vi "InjectApplicationReference.vi"(8 "error in (no error)":errorcluster, 10 "Application":refnum<vi>, 11 "CreateClass In":refnum<class "CreateClass.lvclass">) -> (0 "error out":errorcluster, 3 "CreateClass Out":refnum<class "CreateClass.lvclass">)   [LabVIEW 2020, in "Mermaid.lvlib" / "CreateClass.lvclass"]
uses:
  CreateClass.lvclass
  CreateClass.lvclass/CreateClass.ctl
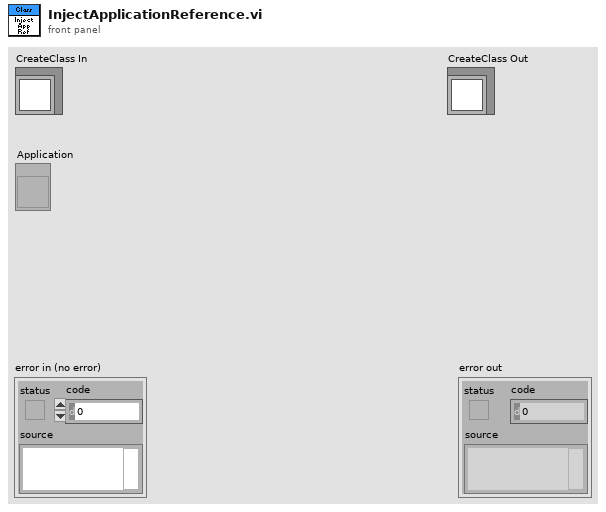
[diagram p1: front panel]
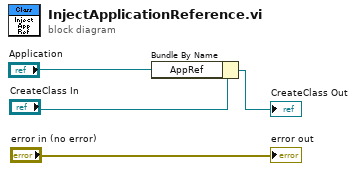
[diagram p0: block diagram]
diagram:
  n1 = Bundle By Name(cluster="CreateClass In", "AppRef"="Application") -> (→"CreateClass Out":refnum<class "CreateClass.lvclass">)
  "error out" <- "error in (no error)"
